vi "Scope Report Event.vi"(8 "error in (no error)":errorcluster, 9 "Event Data":variant, 10 "Scope Events":T1, 11 "Unit_Test_Scope in":refnum<class "Unit_Test_Scope.lvclass">) -> (0 "error out":errorcluster, 3 "Unit_Test_Scope out":refnum<class "Unit_Test_Scope.lvclass">)   [LabVIEW 2020, in "Unit_Test_Scope.lvlib" / "Unit_Test_Scope.lvclass"]
uses:
  Unit_Test_Scope.lvclass
  Actor_Scope/Actor_Scope/Scope_Event.ctl
  Unit_Test_Scope.lvclass/Unit_Test_Scope.ctl
  Actor_Scope/Actor_Scope/Actor_Scope.lvclass
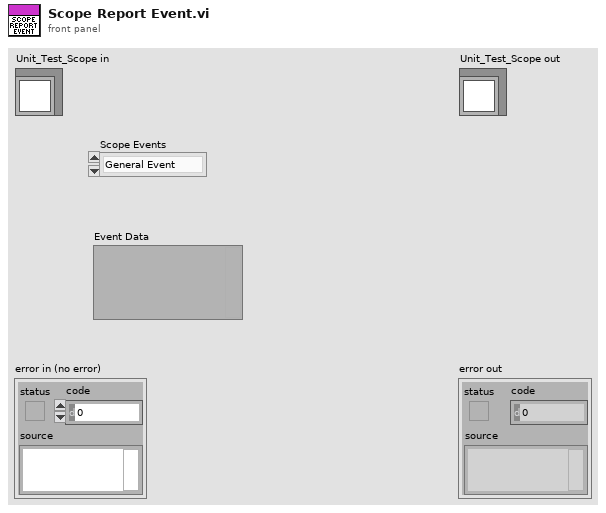
[diagram p1: front panel]
types:
  T1 = typedef "Actor_Scope.lvlib/Actor_Scope.lvclass/Scope_Event.ctl" = enum16{"General Event", "Inited", "Error", "Res Read complete", "Wfm Acq Complete"}
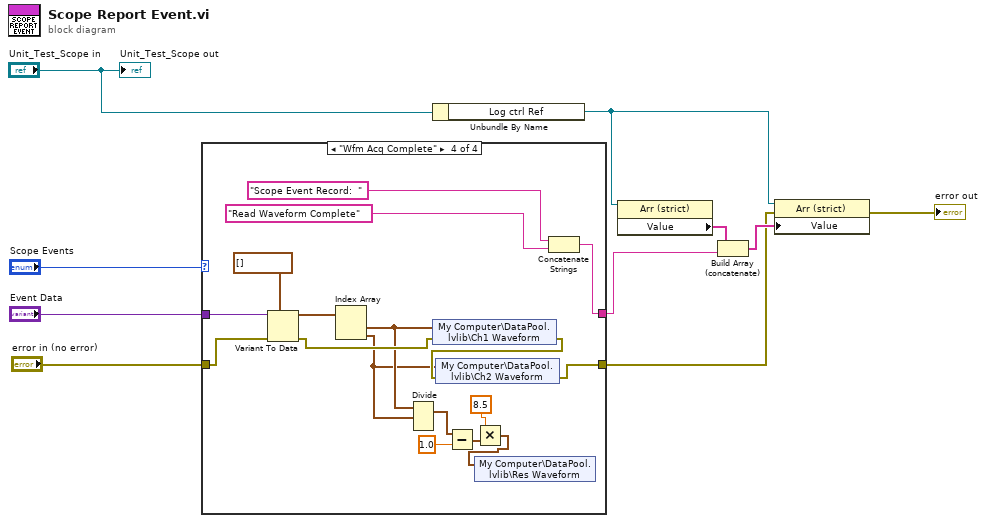
[diagram p0: block diagram]
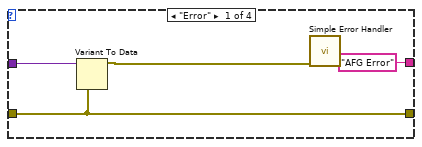
[diagram p2: hidden frame]
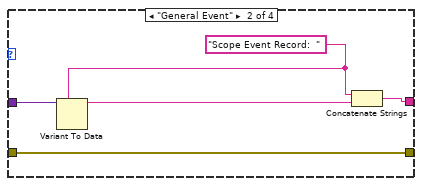
[diagram p3: hidden frame]
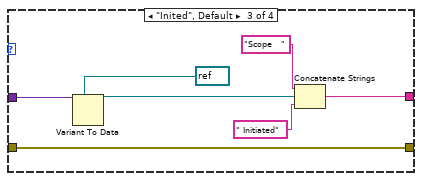
[diagram p4: hidden frame]
diagram:
  n1 = case shown="\"Wfm Acq Complete\"" "Scope Events" {
    tunnel: "Event Data" -> [w13 w17 w26 w40]
    tunnel: "error in (no error)" -> [w14 w19 w21 w39]
    tunnel: [w14 w19 w21 w34] -> w6
    tunnel: ["AFG Error" w15 w20 w41] -> w8
    frame "Error" {
      n2 = Variant To Data(type=w14, Variant=w13) -> (data=w12:errorcluster)  [unwired: 1 in, 1 out]
      n3 = call <vilib>:"Simple Error Handler.vi"("error in (no error)"=w12) -> ()  [unwired: 4 in, 5 out]
    }
    frame "General Event" {
      w18 = "Scope Event Record:  "
      n4 = Variant To Data(type=w18, Variant=w17) -> (data=w16:string)  [unwired: 1 in, 1 out]
      n5 = Concatenate Strings(w18, w16) -> (w15:string)
    }
    frame "Inited", Default {
      n6 = Variant To Data(type=refnum<visa-resource-name> refnum ("VISA resource name"), Variant=w26) -> (data=w24:refnum<visa-resource-name>)  [unwired: 1 in, 1 out]
      n7 = Concatenate Strings("Scope   " ("string"), w24, " Initiated" ("string")) -> (w20:string)
    }
    frame "Wfm Acq Complete" {
      n8 = Variant To Data(error in=w39, type=waveform(dbl)[] [], Variant=w40) -> (data=w37:waveform(dbl)[], error out=w36:errorcluster)
      n9 = Index Array(array=w37) -> (element #1=w28:waveform(dbl), element #2=w27:waveform(dbl))  [unwired: 2 in]
      n10 = Divide(1:w27, 2:w28) -> (0:w33:waveform(dbl))  [unwired: 1 in, 1 out]
      n11 = shared-variable "My Computer\\DataPool.lvlib\\Ch1 Waveform"(w28, error in=w36) -> (error out=w35:errorcluster)
      n12 = shared-variable "My Computer\\DataPool.lvlib\\Ch2 Waveform"(w27, error in=w35) -> (error out=w34:errorcluster)
      n13 = Subtract(x=w33, y=1.0) -> (x-y=w31:waveform(dbl))
      n14 = Multiply(x=8.5, y=w31) -> (x*y=w29:waveform(dbl))
      n15 = shared-variable "My Computer\\DataPool.lvlib\\Res Waveform"(w29) -> ()  [unwired: 1 in, 1 out]
      n16 = Concatenate Strings("Scope Event Record:  ", "Read Waveform Complete" ("string")) -> (w41:string)
    }
  }
  n17 = Unbundle By Name("Unit_Test_Scope in") -> ("Log ctrl Ref"=w7:refnum<vi>)
  n18 = property class="Arr (strict)"(reference=w7) -> ("Value"=w9:string[])  [unwired: 1 in, 2 out]
  n19 = Build Array (concatenate)(w9, w8) -> (w10:string[])
  n20 = property class="Arr (strict)"(reference=w7, error in=w6, "Value"=w10) -> (error out=→"error out":errorcluster)  [unwired: 1 out]
  "Unit_Test_Scope out" <- "Unit_Test_Scope in"
